vi "Flywheel_Globals.vi"() -> ()   [LabVIEW 2019]
panel:
  in  "Flywheel_Left":string="Flywheel_Left"
  in  "Flywheel_Right":string
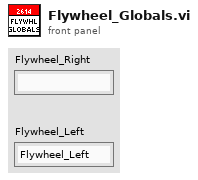
[diagram p1: front panel]
diagram:
